vi "Write serialize_.vi"(8 "error in (no error)":errorcluster, 10 "serialize?":bool, 11 "Update Serialize Waverform CMD in":refnum<class "Update Serialize Waverform CMD.lvclass">) -> (0 "error out":errorcluster, 3 "Update Serialize Waverform CMD out":refnum<class "Update Serialize Waverform CMD.lvclass">)   [LabVIEW 2017, in "gPAS Library.lvlib" / "Update Serialize Waverform CMD.lvclass"]
uses:
  Update Serialize Waverform CMD.lvclass
  Update Serialize Waverform CMD.lvclass/Update Serialize Waverform CMD.ctl
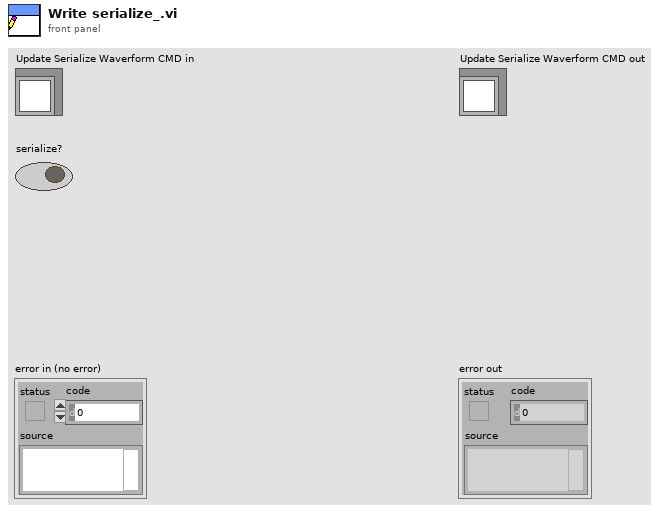
[diagram p1: front panel]
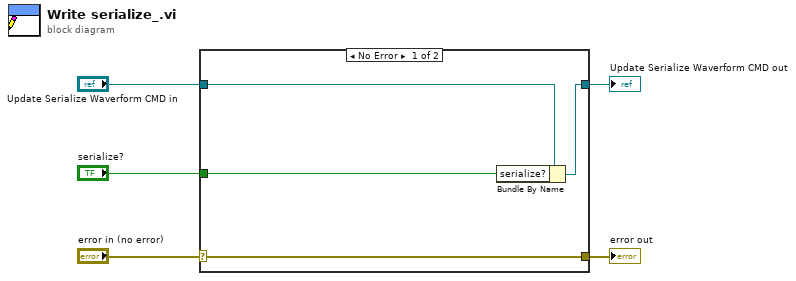
[diagram p0: block diagram]
diagram:
  n1 = case shown="No Error" "error in (no error)" {
    selector: "error in (no error)" -> [w9 w10]
    tunnel: [w9 w10] -> w4
    tunnel: [w7 w11] -> w2
    tunnel: "Update Serialize Waverform CMD in" -> [w8 w11]
    tunnel: "serialize?" -> [w6 _]
    frame No Error {
      n2 = Bundle By Name(cluster=w8, "serialize?"=w6) -> (w7:refnum<class "Update Serialize Waverform CMD.lvclass">)
    }
    frame Error {
    }
  }
  "error out" <- w4
  "Update Serialize Waverform CMD out" <- w2
